vi "Histogram_fit.vi"() -> ()   [LabVIEW 2014]
doc: "This program takes the data from the count rate VI(the data from the gieger counter experiment) and creates a histogram and checks to see if it obeys the Poisson distribution. The values for bin size and where to set the index are not user controlled from the interface because the histrogram VI does not allow changing these parameters easily, hence they must be set in the block diagram. Data is imported from a spread sheet, placed in a histogram and compared with a Poisson distribution."
uses:
  <vilib>/gmath/SpecialFunctions.llb/Factorial.vi
  <vilib>/Utility/file.llb/Read From Spreadsheet File (DBL).vi
  <vilib>/imath/engines/lvmath2/RunTimeEngine/Managers/WorkSpace/UID Generator.vi
  <vilib>/imath/engines/lvmath2/RunTimeEngine/BuiltInFunctions/linramp/NIMS_linramp.vi
  <vilib>/imath/engines/lvmath2/RunTimeEngine/RunTimeType/NIMS_RunTimeType_From StrictType (excl LVString).vi
  <instcachedir>/0/NIMS_RunTimeType_From StrictType (excl LVString)_15A5391EEA9C4AACB9955AC755B83D29.lvgen/NIMS_RunTimeType_From StrictType (excl LVString)_15A5391EEA9C4AACB9955AC755B83D29_000.vi
  <vilib>/imath/engines/lvmath2/RunTimeEngine/LocalVariableDefStatement/MC_LocalVariableDefStatement_Display.vi
  <vilib>/imath/engines/lvmath2/RunTimeEngine/Managers/SymbolTable/Clear UID.vi
  <vilib>/imath/engines/lvmath2/RunTimeEngine/NodeEndStatement/NIMS_NodeEndStatement_Output.vi
  <instcachedir>/0/NIMS_NodeEndStatement_Output_53EC0D466D134D7ABD903AC30B43404B.lvgen/NIMS_NodeEndStatement_Output_53EC0D466D134D7ABD903AC30B43404B_005.vi
  <vilib>/imath/engines/lvmath2/RunTimeEngine/ErrorHandling/NIMS_Finalize Error.vi
  <vilib>/imath/engines/lvmath2/RunTimeEngine/ArithmeticOperatorToken/NIMS_ArithmeticOperator_power(S).vi
  <instcachedir>/0/NIMS_ArithmeticOperator_power(S)_CAFE680B12A64A3A8F5E28A20C679B7D.lvgen/NIMS_ArithmeticOperator_power(S)_CAFE680B12A64A3A8F5E28A20C679B7D_015.vi
  <vilib>/imathl/engines/lvmath/Functions/Error Handling/Create Error.vi
  <vilib>/imath/engines/lvmath2/RunTimeEngine/ArithmeticOperatorToken/NIMS_ArithmeticOperator_rightdiv(C,C).vi
  <instcachedir>/0/NIMS_ArithmeticOperator_rightdiv(C,C)_B4CE00C486B54A9B9073334614CFE190.lvgen/NIMS_ArithmeticOperator_rightdiv(C,C)_B4CE00C486B54A9B9073334614CFE190_000.vi
  <instcachedir>/0/NIMS_NodeEndStatement_Output_53EC0D466D134D7ABD903AC30B43404B.lvgen/NIMS_NodeEndStatement_Output_53EC0D466D134D7ABD903AC30B43404B_000.vi
  <vilib>/imath/engines/lvmath2/RunTimeEngine/Managers/SymbolTable/NIMS_WorkSpace.lvlib
  <vilib>/gmath/NI_Gmath.lvlib
panel:
  out "Histogram":cluster{"y":dbl[], "output":dbl[]}[](graph)=[{"y"=[35.0, 37.89473684210526, 40.78947368421053, 43.68421052631579, 46.578947368421055, 49.473684210526315, 52.36842105263158, 55.26315789473684, 58.1578947368421, 61.05263157894737, 63.94736842105263, 66.84210526315789, 69.73684210526316, 72.63157894736842, 75.52631578947368, 78.42105263157895, 81.3157894736842, 84.21052631578948, 87.10526315789474, 90.0], "output"=[0.0, 1.0, 2.0, 1.0, 13.0, 16.0, 32.0, 28.0, 56.0, 41.0, 38.0, 19.0, 27.0, 15.0, 4.0, 2.0, 5.0, 0.0, 0.0, 0.0]}, {"y"=[35.0, 36.0, 37.0, 38.0, 39.0, 40.0, 41.0, 42.0, 43.0, 44.0, 45.0, 46.0, 47.0, 48.0, 49.0, 50.0, 51.0, 52.0, 53.0, 54.0, 55.0, 56.0, 57.0, 58.0, 59.0, 60.0, 61.0, 62.0, 63.0, 64.0, 65.0, 66.0, 67.0, 68.0, 69.0, 70.0, 71.0, 72.0, 73.0, 74.0, 75.0, 76.0, 77.0, 78.0, 79.0, 80.0, 81.0, 82.0, 83.0, 84.0, 85.0, 86.0, 87.0, 88.0, 89.0, 90.0], "output"=[0.14567740642834123, 0.2427956773805663, 0.39372272007660125, 0.621667452752522, 0.9564114657731012, 1.434617198659678, 2.0994398029165815, 2.9991997184522283, 4.18492983970086, 5.706722508682935, 7.608963344910503, 9.924734797709535, 12.669874209841831, 15.83734276230213, 19.392664606900926, 23.271197528280872, 27.377879445036825, 31.5898608981191, 35.762106677115604, 39.735674085684735, 43.34800809347381, 46.444294385864325, 48.888730932489665, 50.57454924050605, 51.43174499034462, 51.431744990345564, 50.58860162984759, 48.95671125469072, 46.625439290182506, 43.71134933454566, 40.348937847272516, 36.680852588429175, 32.848524706057525, 28.983992387697516, 25.20347164147585, 21.602975692693374, 18.256035796642102, 15.21336316386826, 12.50413410728957, 10.138487114018467, 8.110789691214695, 6.403255019379957, 4.989549365750566, 3.8381148967311662, 2.915023972201022, 2.1862679791507444, 1.6194577623338684, 1.1849690943906237, 0.8566041646197192, 0.6118601175855077, 0.43190125947214325, 0.3013264600968411, 0.20781135179092278, 0.14168955803926417, 0.0955210503635479, 0.06368070024236464]}]
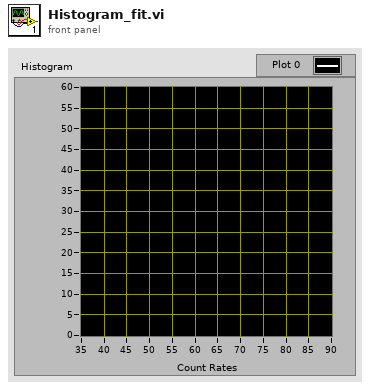
[diagram p1: front panel]
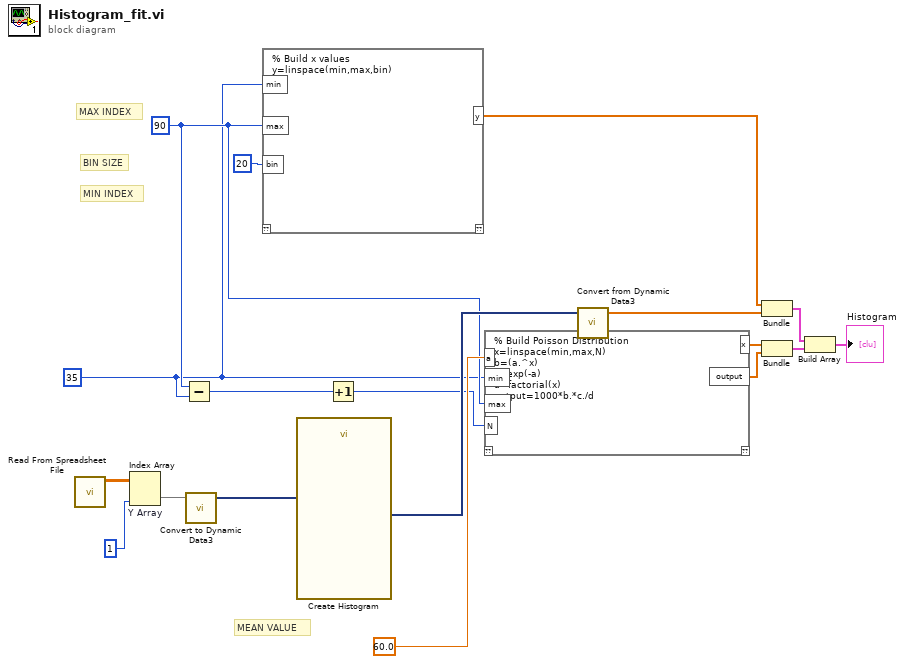
[diagram p0: block diagram]
diagram:
  w2 = 90 ("stop")
  w1 = 35 ("start")
  # "BIN SIZE"
  # "MAX INDEX"
  # "MIN INDEX"
  # "MEAN VALUE"
  n1 = call-poly <vilib>:"Read From Spreadsheet File.vi"() -> ("all rows"=w18:dbl[][])  [unwired: 7 in, 4 out]
  n2 = Index Array "Y Array"(array=w18, index (col)=1 ("disabled index (col)")) -> (element=w16:dbl[])  [unwired: 1 in]
  n3 = Subtract(x=w2, y=w1) -> (x-y=w4:i32)
  n4 = call "Convert to Dynamic Data3"("Array"=w16) -> ("Dynamic Data Type"=w15:dynamicdata)  [unwired: 3 in]
  n5 = mathscript code="% Build x values\ny=linspace(min,max,bin)"("min"=w1, "max"=w2, "bin"=20 ("N")) -> ("y"=w9:dbl[])  [unwired: 1 in, 1 out]
  n6 = call "Create Histogram"("Signal"=w15) -> ("Histogram"=w14:dynamicdata)  [unwired: 9 in, 1 out]
  n7 = Increment(x=w4) -> (x+1=w3:i32)
  n8 = mathscript code="% Build Poisson Distribution\nx=linspace(min,max,N)\nb=(a.^x)\nc=exp(-a)\nd=factorial(x)\noutput=1000*b.*c./d"("a"=60.0, "min"=w1, "max"=w2, "N"=w3) -> ("output"=w5:cdb[], "x"=w6:dbl[])  [unwired: 1 in, 1 out]
  n9 = call "Convert from Dynamic Data3"("Dynamic Data Type"=w14) -> ("Array"=w11:dbl[])  [unwired: 3 in]
  n10 = Bundle("y"=w9, "Array"=w11) -> (w7:cluster{"y":dbl[], "Array":dbl[]})  [unwired: 1 in]
  n11 = Bundle("x"=w6, "output"=w5) -> (w8:cluster{"x":dbl[], "output":cdb[]})  [unwired: 1 in]
  n12 = Build Array(w7, w8) -> (→"Histogram":cluster{"x":dbl[], "output":cdb[]}[])
